vi "PWŚG_Projekt.vi"() -> ()   [LabVIEW 2023]
panel:
  out "Twój wiek to:":dbl
  in  "Ile masz lat?":dbl
  in  "Jaka jest twoja plec?":bool
  out "Twoja plec:":string
  out "Twój wynik to:":dbl
  in  "Jak często w ciągu ostatniego miesiąca czułeś/aś, że nie możesz przezwyciężyć narastających trudności?":dbl
  in  "Jak często w ciągu ostatniego miesiąca złościłeś/aś się, ponieważ nie miałeś/aś wpływu na\nto co się zdarzyło?":dbl
  in  "Jak często w ciągu ostatniego miesiąca czułeś/aś, że nic wszystko ci wychodzi?":dbl
  in  "Jak często w ciągu ostatniego miesiąca nie potrafiłeś/aś opanować swoje rozdrażnienie?":dbl
  in  "Jak często w ciągu ostatniego miesiąca stwierdzałeś/aś, że nie radzisz sobie ze wszystkimi\nobowiązkami?":dbl
  in  "Jak często w ciągu ostatniego miesiąca czułeś/aś, że sprawy nie układają się po twojej myśli?":dbl
  in  "Jak często w ciągu ostatniego miesiąca byłeś/aś przekonany/a, że nie jesteś w stanie poradzić\nsobie z problemami osobistymi?":dbl
  in  "Jak często w ciągu ostatniego miesiąca odczuwałeś/aś zdenerwowanie i napięcie?":dbl
  in  "Jak często w ciągu ostatniego miesiąca czułeś/aś, że ważne sprawy w twoim życiu\nwymykają ci się spod kontroli?":dbl
  in  "Jak często w ciągu ostatniego miesiąca byłeś/aś zdenerwowany/a, ponieważ zdarzyło się\ncoś niespodziewanego?":dbl
  # "Pytania zawarte w tej skali dotyczą Twoich myśli i odczuć związanych z doświadczanymi w ostatnim\nmiesiącu zdarzeniami. W każdym pytaniu należy wskazać – jak często myślałeś/aś i odczuwałeś/aś w podany sposób. Mimo znacznych podobieństw są to różne pytania i każde z nich należy traktować oddzielnie. Najlepiej na każde pytanie odpowiadać w miarę szybko, wybierając tę odpowiedź, która wydaje się\nnajbardziej trafna.\nPrzy każdym pytaniu należy wpisać do kratki z prawej strony odpowiednią cyfrę, zgodnie z podanym\nponiżej znaczeniem:"
  # "0 = nigdy\n1 = prawie nigdy\n2 = czasem\n3 = dość często\n4 = bardzo często"
  # "Mezczyzna"
  # "Kobieta"
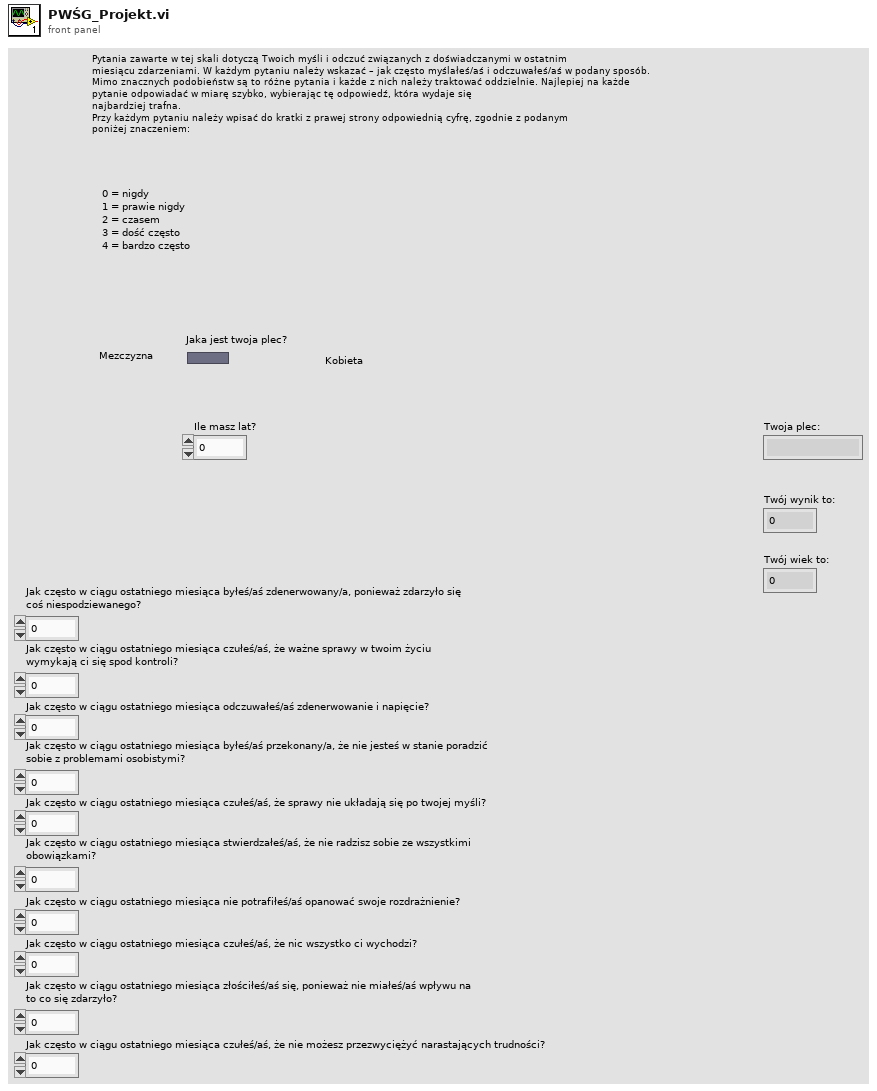
[diagram p1: front panel]
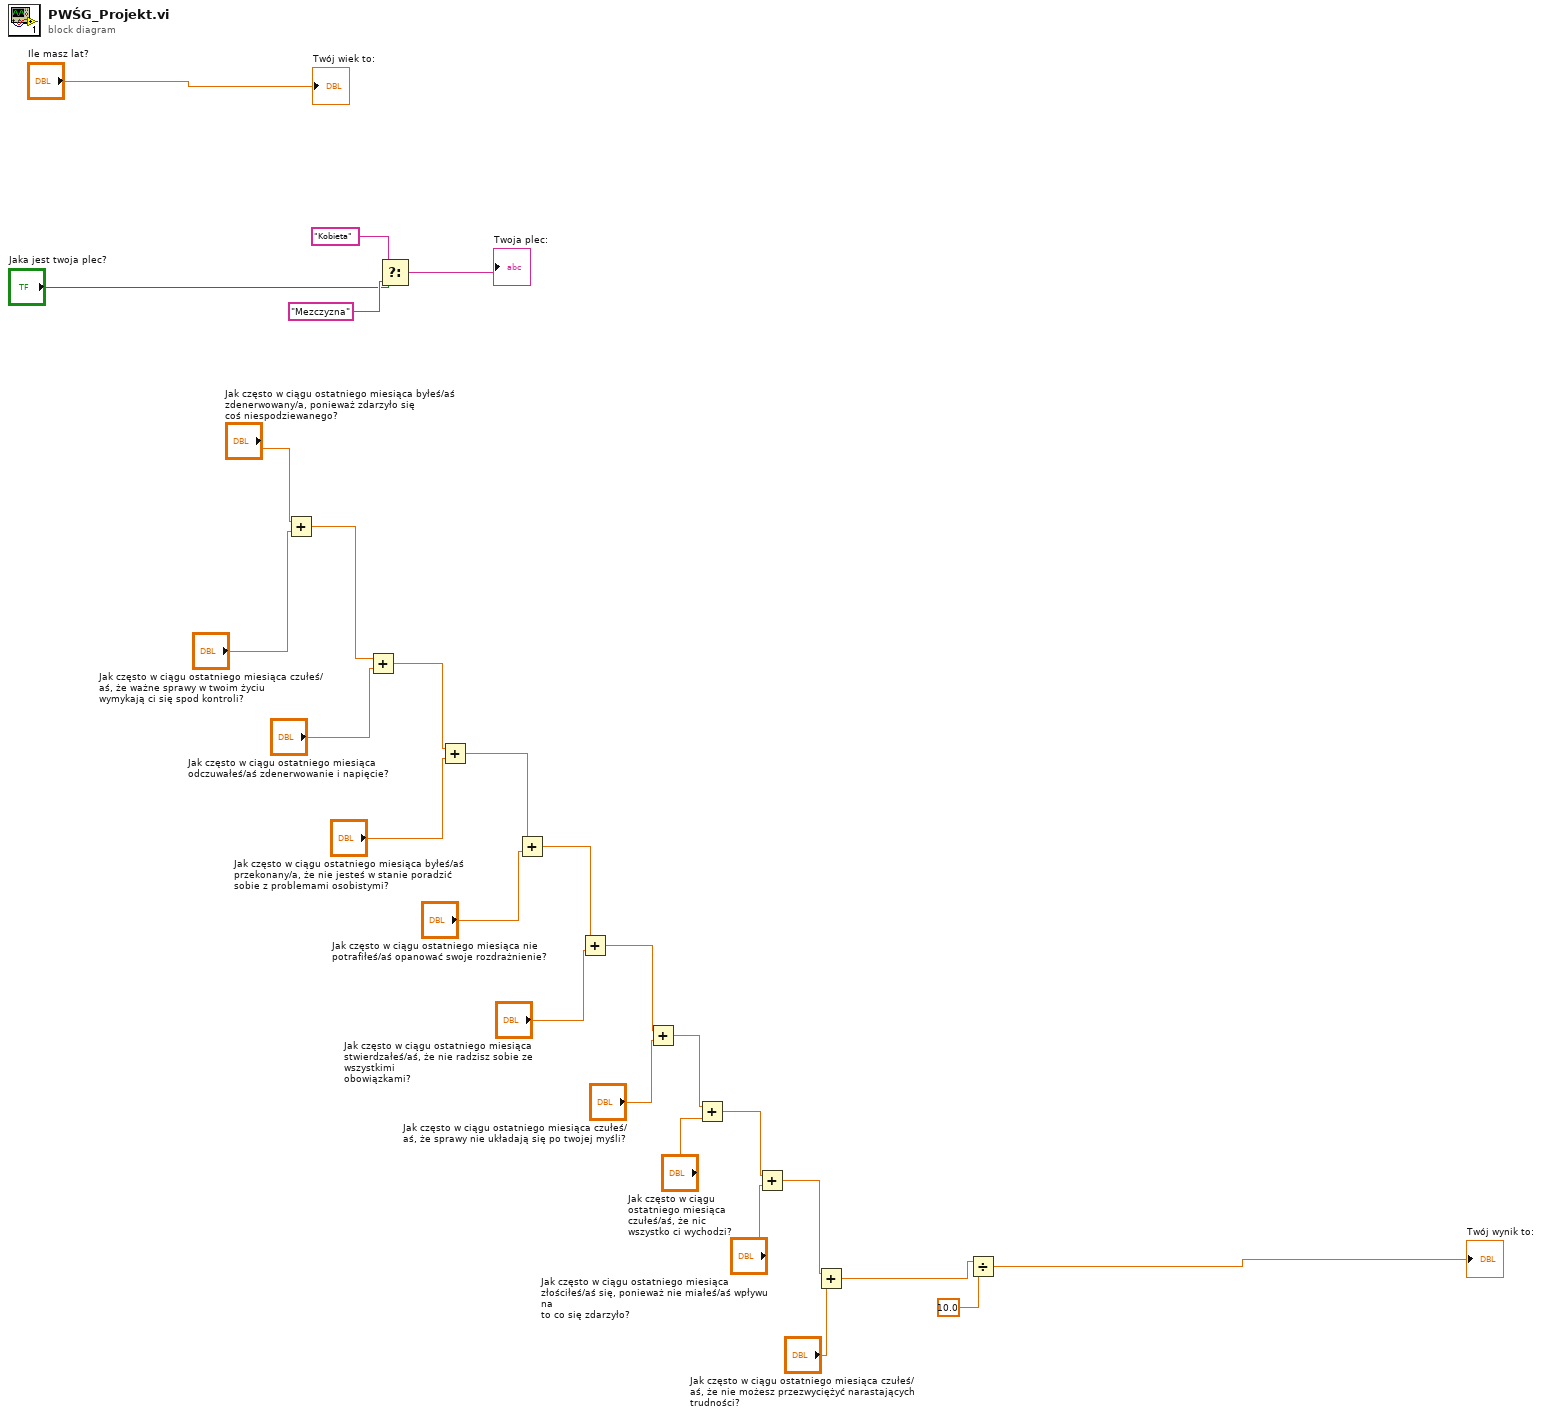
[diagram p0: block diagram]
diagram:
  n1 = Add(x="Jak często w ciągu ostatniego miesiąca byłeś/aś zdenerwowany/a, ponieważ zdarzyło się\ncoś niespodziewanego?", y="Jak często w ciągu ostatniego miesiąca czułeś/aś, że ważne sprawy w twoim życiu\nwymykają ci się spod kontroli?") -> (x+y=w24:dbl)
  n2 = Add(x=w24, y="Jak często w ciągu ostatniego miesiąca odczuwałeś/aś zdenerwowanie i napięcie?") -> (x+y=w22:dbl)
  n3 = Select(t="Kobieta", s="Jaka jest twoja plec?", f="Mezczyzna") -> (s? t:f=→"Twoja plec:":string)
  n4 = Add(x=w22, y="Jak często w ciągu ostatniego miesiąca byłeś/aś przekonany/a, że nie jesteś w stanie poradzić\nsobie z problemami osobistymi?") -> (x+y=w20:dbl)
  n5 = Add(x=w20, y="Jak często w ciągu ostatniego miesiąca nie potrafiłeś/aś opanować swoje rozdrażnienie?") -> (x+y=w18:dbl)
  n6 = Add(x=w18, y="Jak często w ciągu ostatniego miesiąca stwierdzałeś/aś, że nie radzisz sobie ze wszystkimi\nobowiązkami?") -> (x+y=w15:dbl)
  n7 = Add(x=w15, y="Jak często w ciągu ostatniego miesiąca czułeś/aś, że sprawy nie układają się po twojej myśli?") -> (x+y=w14:dbl)
  n8 = Add(x=w14, y="Jak często w ciągu ostatniego miesiąca czułeś/aś, że nic wszystko ci wychodzi?") -> (x+y=w12:dbl)
  n9 = Add(x=w12, y="Jak często w ciągu ostatniego miesiąca złościłeś/aś się, ponieważ nie miałeś/aś wpływu na\nto co się zdarzyło?") -> (x+y=w10:dbl)
  n10 = Add(x=w10, y="Jak często w ciągu ostatniego miesiąca czułeś/aś, że nie możesz przezwyciężyć narastających trudności?") -> (x+y=w8:dbl)
  n11 = Divide(x=w8, y=10.0) -> (x/y=→"Twój wynik to:":dbl)
  "Twój wiek to:" <- "Ile masz lat?"
